vi "cumplimiento.vi"(8 "error in (no error)":errorcluster, 11 "Prueba04 in":refnum<class "Prueba05.lvclass">) -> (0 "error out":errorcluster, 3 "Prueba04 out":refnum<class "Prueba05.lvclass">)   [LabVIEW 2019, in "Prueba05.lvclass"]
uses:
  Prueba05.lvclass
  Prueba05.lvclass/Prueba05.ctl
panel:
  out "cumpimiento":string
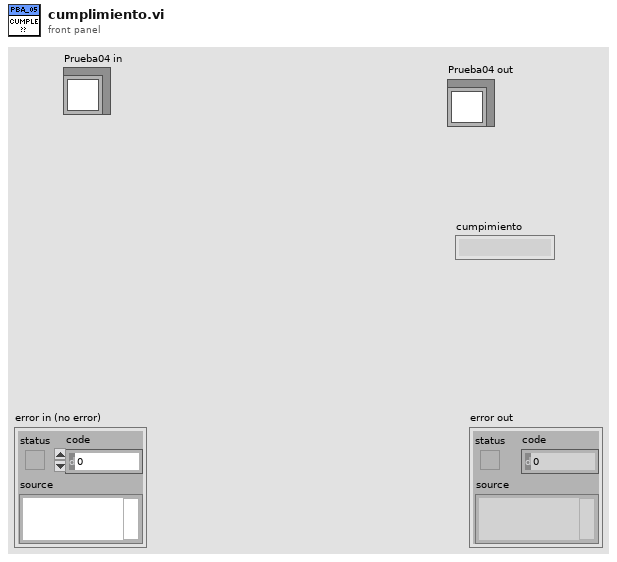
[diagram p1: front panel]
types:
  T1 = cluster{"Medido":dbl, "error":dbl, "Ref":dbl, "Incert_exp":dbl, "Tol+":dbl, "Tol-":dbl, "fila":i32}
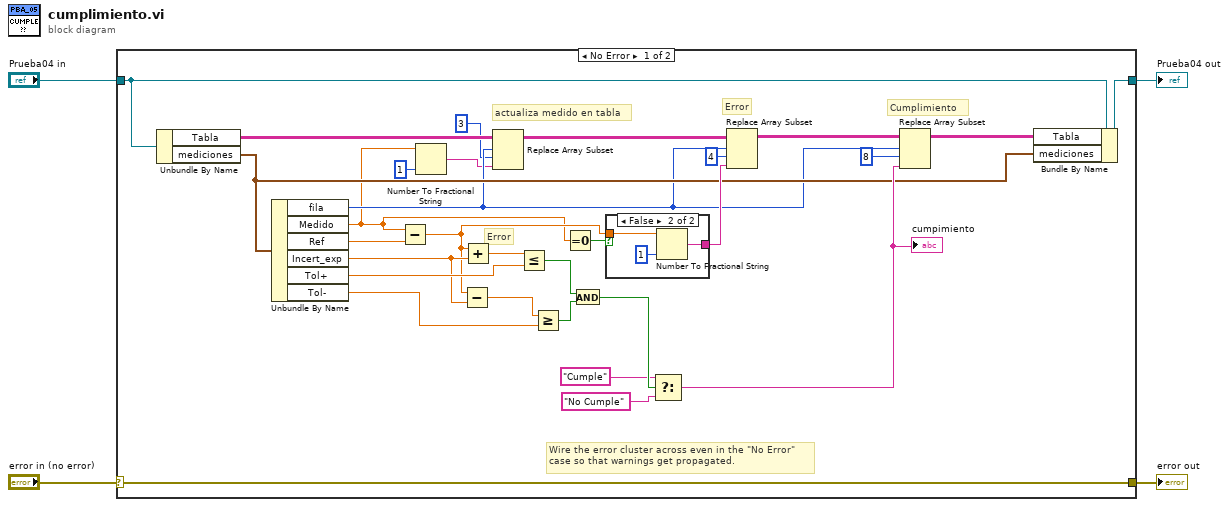
[diagram p0: block diagram]
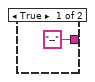
[diagram p2: hidden frame]
diagram:
  n1 = case shown="No Error" "error in (no error)" {
    selector: "error in (no error)" -> [w34 w40]
    tunnel: [w34 w40] -> w3
    tunnel: [w15 w39] -> w2
    tunnel: "Prueba04 in" -> [w13 w39]
    frame No Error {
      # "actualiza medido en tabla"
      # "Cumplimiento"
      # "Error"
      # "Error"
      # "Wire the error cluster across even in the \"No Error\"\ncase so that warnings get propagated."
      n2 = Unbundle By Name(w13) -> ("Tabla"=w12:string[][], "mediciones"=w11:T1)
      n3 = Unbundle By Name(w11) -> ("fila"=w9:i32, "Medido"=w7:dbl, "Ref"=w26:dbl, "Incert_exp"=w24:dbl, "Tol+"=w25:dbl, "Tol-"=w23:dbl)
      n4 = Subtract(x=w7, y=w26) -> (x-y=w16:dbl)
      n5 = Number To Fractional String(number=w7, precision (6)=i16 1) -> (F-format string=w6:string)  [unwired: 2 in]
      n6 = Subtract(x=w16, y=w24) -> (x-y=w30:dbl)
      n7 = Add(x=w16, y=w24) -> (x+y=w33:dbl)
      n8 = Replace Array Subset(array=w12, new element=w6, index (row)=w9, index (col)=3 ("disabled index (col)")) -> (w10:string[][])
      n9 = Less Or Equal?(x=w33, y=w25) -> (x <= y?=w32:bool)
      n10 = Greater Or Equal?(x=w30, y=w23) -> (x >= y?=w31:bool)
      n11 = Equal To 0?(x=w7) -> (x = 0?=w17:bool)
      n12 = And(x=w32, y=w31) -> (x .and. y?=w29:bool)
      n13 = case shown="False" w17 {
        tunnel: w16 -> [_ w38]
        tunnel: ["--" w36] -> w18
        frame True {
        }
        frame False {
          n14 = Number To Fractional String(number=w38, precision (6)=i16 1) -> (F-format string=w36:string)  [unwired: 2 in]
        }
      }
      n15 = Select(t="Cumple", s=w29, f="No Cumple") -> (s? t:f=w22:string)
      "cumpimiento" <- w22
      n16 = Replace Array Subset(array=w10, new element=w18, index (row)=w9, index (col)=4 ("disabled index (col)")) -> (w20:string[][])
      n17 = Replace Array Subset(array=w20, new element=w22, index (row)=w9, index (col)=8 ("index (row)")) -> (w14:string[][])
      n18 = Bundle By Name(cluster=w13, "Tabla"=w14, "mediciones"=w11) -> (w15:refnum<class "Prueba05.lvclass">)
    }
    frame Error {
    }
  }
  "error out" <- w3
  "Prueba04 out" <- w2
